vi "Teleop.vi"() -> ()   [LabVIEW 2016]
doc: "This VI is called for each TeleOp packet received from the DS where the robot is not disabled. It is often used to read from the joysticks and update I/O or to update setpoints for timed control loops. It should complete and return within 20 milliseconds or it may miss DS packets."
uses:
  <vilib>/Rock Robotics/WPI/Utilities/WPI_GetSetVariantRefNum.vi
  External/2ndContollerStatus.vi
  External/External.lvlib
panel:
  out "Angle":u16
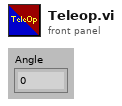
[diagram p1: front panel]
types:
  T1 = enum16{"A", "B", "X", "Y", "LB", "RB", "Back", "Start"}
  T2 = typedef "WPI_JoystickDevRef.ctl" = cluster{"Device":T3}
  T3 = typedef "WPI_JoystickDeviceEnum.ctl" = enum16{"USB 0", "USB 1", "USB 2", "USB 3", "USB 4", "USB 5"}
  T4 = typedef "WPI_RobotDriveDevRef.ctl" = cluster{"DevStatus":errorcluster, "Motors[]":T5[], "Square Inputs":bool, "Max Output":dbl}
  T5 = typedef "WPI_MotorControlDeviceRef.ctl" = cluster{"DeviceStatus":errorcluster, "Type":T6, "PWM":cluster{"PWM Channel":T7, "DeadBand":T8}, "CAN":cluster{"Device Number":u8, "SetOutput VI Ref":variant, "GetOutput VI Ref":variant, "Enable VI Ref":variant, "Disable VI Ref":variant, "Data":variant}, "Invert":bool}
  T6 = typedef "WPI_MotorControlType.ctl" = enum16{"PWM", "CAN"}
  T7 = typedef "FPGA_DIOPWMChannel.ctl" = enum8{"PWM 0", "PWM 1", "PWM 2", "PWM 3", "PWM 4", "PWM 5", "PWM 6", "PWM 7", "PWM 8", "PWM 9", "PWM MXP 0", "PWM MXP 1", "PWM MXP 2", "PWM MXP 3", "PWM MXP 4", "PWM MXP 5", "PWM MXP 6", "PWM MXP 7", "PWM MXP 8", "PWM MXP 9", "Invalid"}
  T8 = typedef "WPI_PWMDeadband.ctl" = cluster{"Name":string, "maxPositivePwm":i32, "minPositivePwm":i32, "centerPwm":i32, "maxNegativePwm":i32, "minNegativePwm":i32, "angularRange":u16}
  T9 = typedef "WPI_ServoDeviceRef.ctl" = cluster{"DeviceStatus":errorcluster, "PWM Channel":T7, "DeadBand":T8}
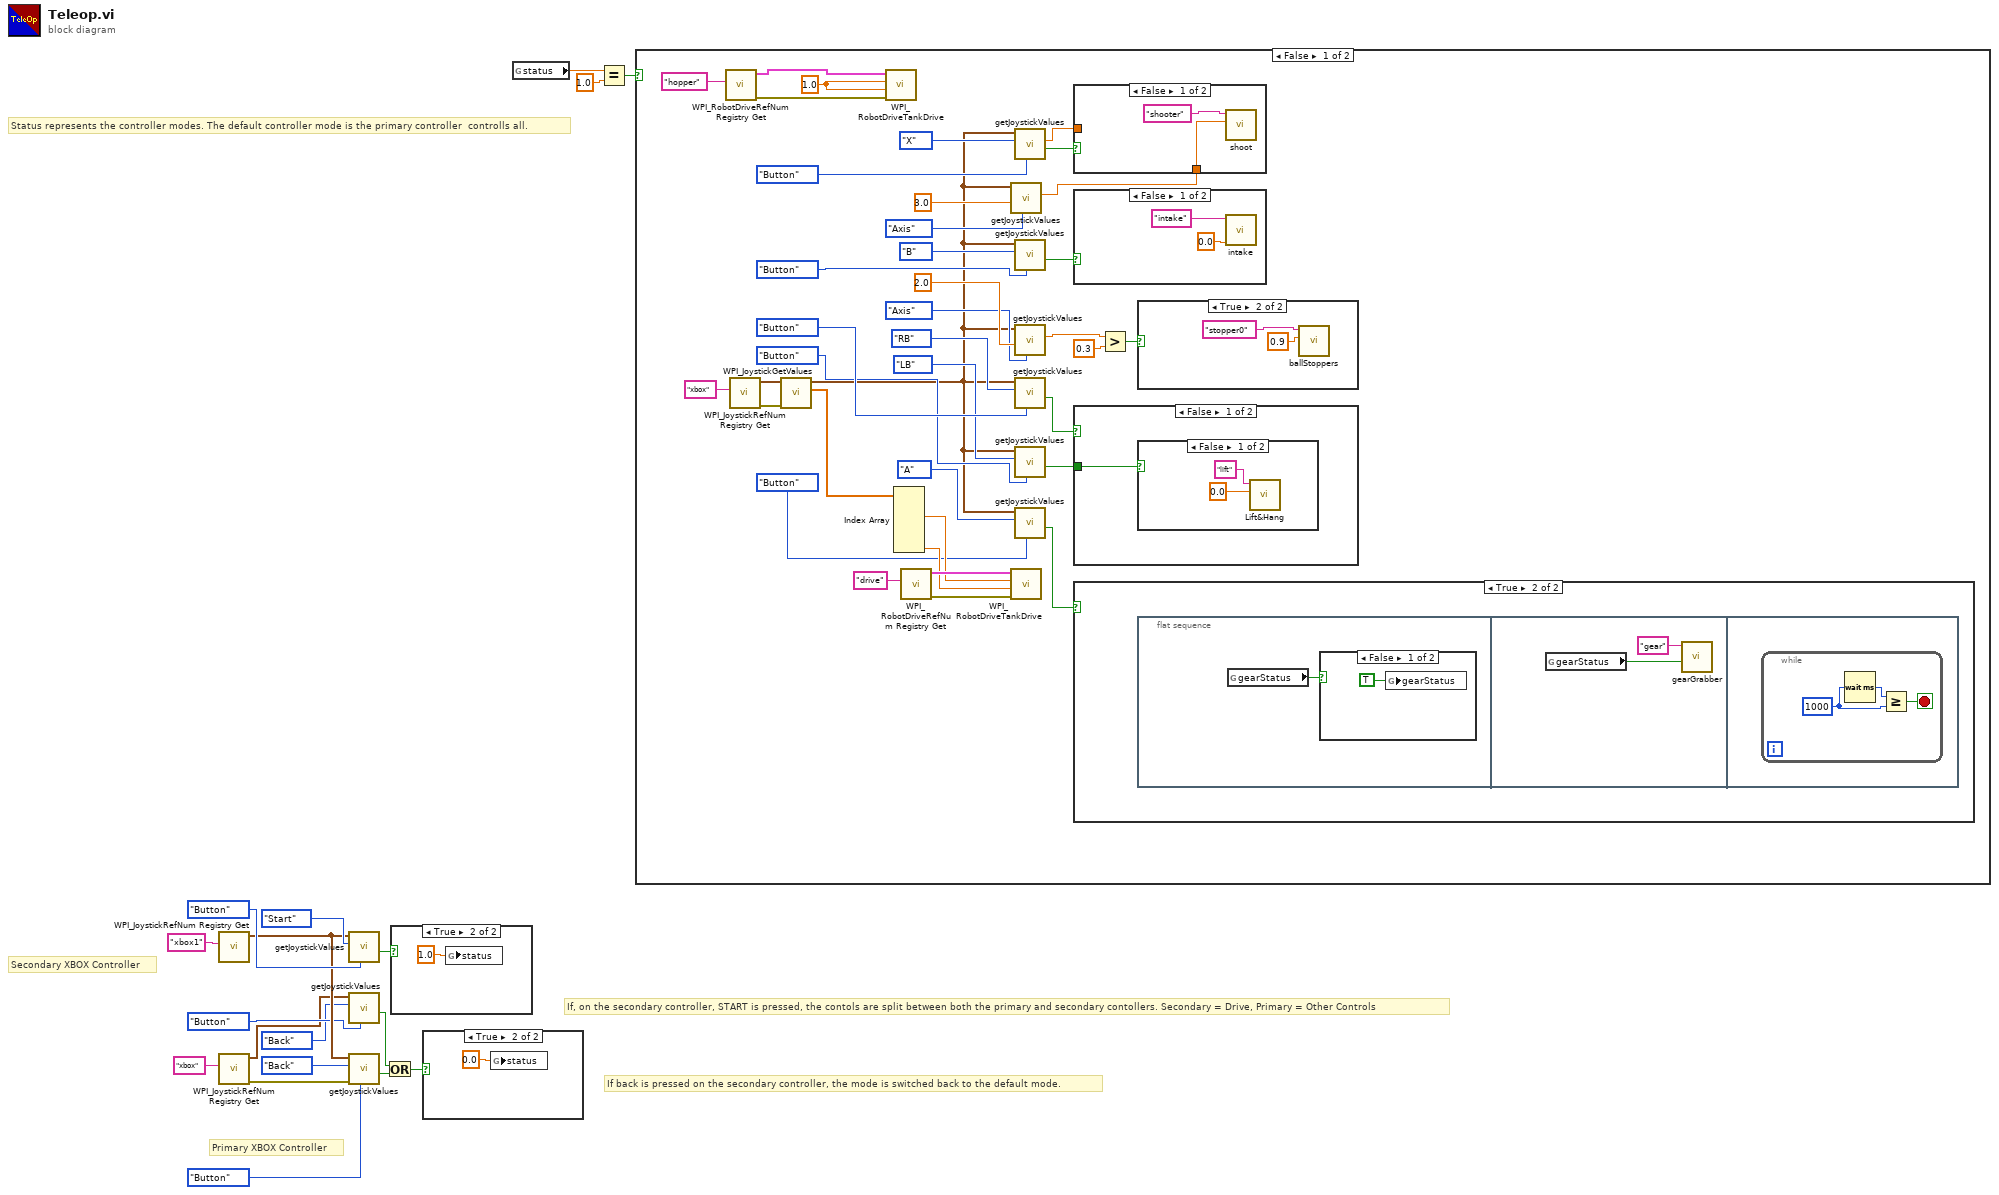
[diagram p0: block diagram]
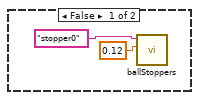
[diagram p2: hidden frame]
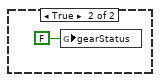
[diagram p4: hidden frame]
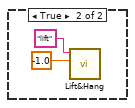
[diagram p5: hidden frame]
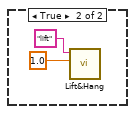
[diagram p6: hidden frame]
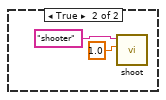
[diagram p7: hidden frame]
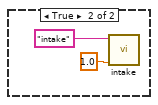
[diagram p8: hidden frame]
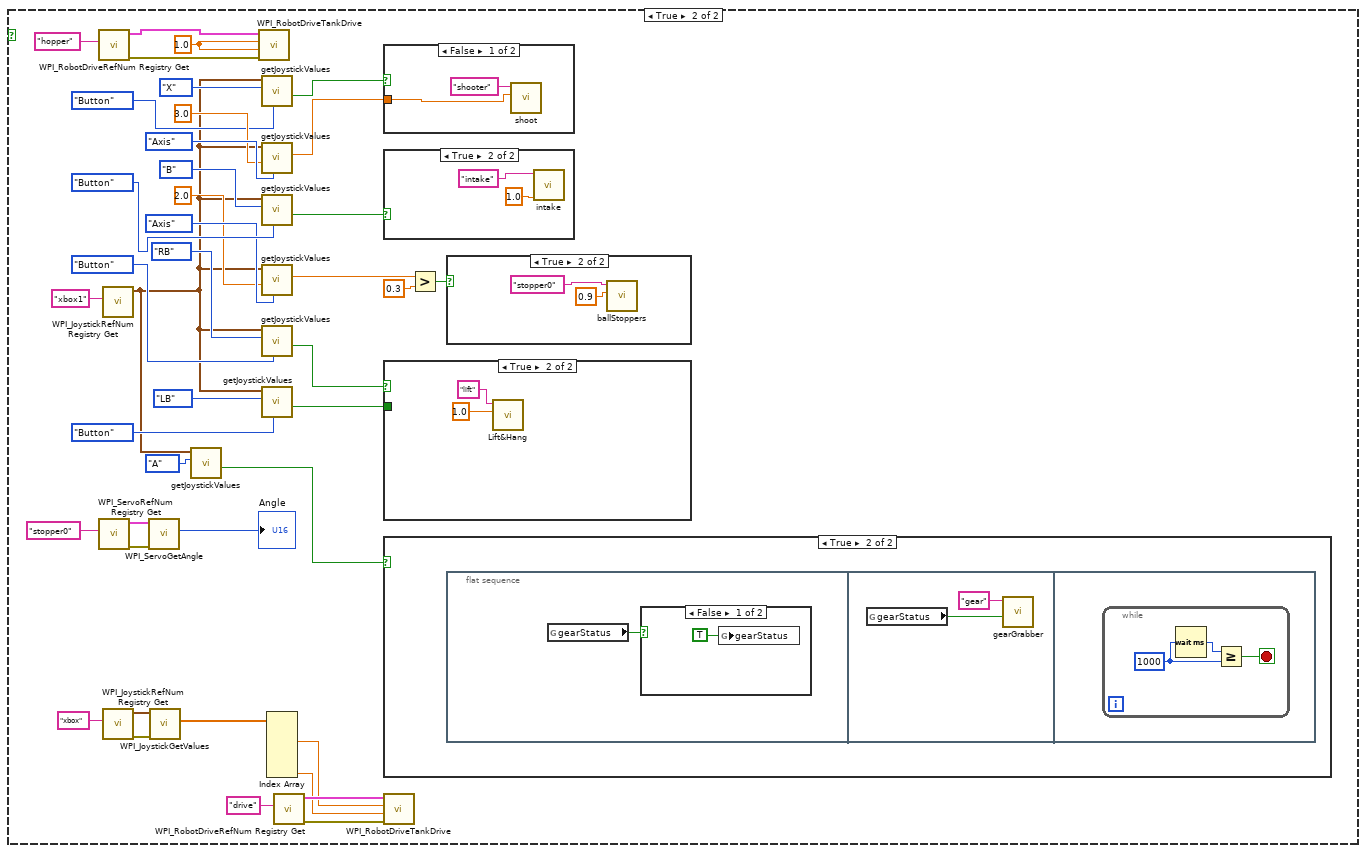
[diagram p9: hidden frame]
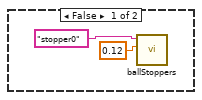
[diagram p10: hidden frame]
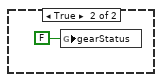
[diagram p12: hidden frame]
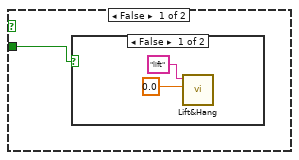
[diagram p13: hidden frame]
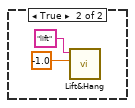
[diagram p14: hidden frame]
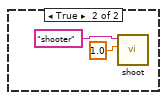
[diagram p15: hidden frame]
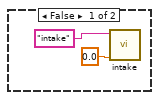
[diagram p16: hidden frame]
diagram:
  # "Secondary XBOX Controller"
  # "Primary XBOX Controller"
  # "If back is pressed on the secondary controller, the mode is switched back to the default mode."
  # "If, on the secondary controller, START is pressed, the contols are split between both the primary and secondary contollers. Secondary = Drive, Primary = Other Controls"
  # "Status represents the controller modes. The default controller mode is the primary controller  controlls all."
  n1 = call <vilib>:"WPI_JoystickRefNum Registry Get.vi"("refnum name"="xbox1" ("xbox1")) -> ("JoystickDevRef"=w13:T2)  [unwired: 9 in, 1 out]
  n2 = call <vilib>:"WPI_JoystickRefNum Registry Get.vi"("refnum name"="xbox" ("xbox")) -> ("error out"=w12:errorcluster, "JoystickDevRef"=w2:T2)  [unwired: 9 in]
  n3 = call "getJoystickValues.vi"("Mode"=enum16{"Axis", "Button"}."Button", "buttonType"=T1."Start", "JoystickDevRef"=w13) -> ("Button Pressed"=w5:bool)  [unwired: 5 in, 3 out]
  n4 = call "getJoystickValues.vi"("Mode"=enum16{"Axis", "Button"}."Button", "buttonType"=T1."Back", "JoystickDevRef"=w2) -> ("Button Pressed"=w3:bool)  [unwired: 5 in, 3 out]
  n5 = call "getJoystickValues.vi"("Mode"=enum16{"Axis", "Button"}."Button", "error in (no error)"=w12, "buttonType"=T1."Back", "JoystickDevRef"=w13) -> ("Button Pressed"=w4:bool)  [unwired: 4 in, 3 out]
  n6 = Or(x=w3, y=w4) -> (x .or. y?=w1:bool)
  n7 = case shown="True" w5 {
    frame False {
    }
    frame True {
      n8 = global write "2ndContollerStatus.vi" "status"(1.0 ("status")) -> ()
    }
  }
  n9 = case shown="True" w1 {
    frame False {
    }
    frame True {
      n10 = global write "2ndContollerStatus.vi" "status"(0.0 ("status")) -> ()
    }
  }
  n11 = global read "2ndContollerStatus.vi" "status"() -> (w11:dbl)
  n12 = Equal?(x=w11, y=1.0) -> (x = y?=w8:bool)
  n13 = case shown="False" w8 {
    frame False {
      w33 = 1.0 ("Left axis value")
      n14 = call <vilib>:"WPI_RobotDriveRefNum Registry Get.vi"("refnum name"="hopper") -> ("error out"=w35:errorcluster, "RobotDriveDevRef"=w36:T4)  [unwired: 9 in]
      n15 = call <vilib>:"WPI_JoystickRefNum Registry Get.vi"("refnum name"="xbox") -> ("error out"=w44:errorcluster, "JoystickDevRef"=w43:T2)  [unwired: 9 in]
      n16 = call <vilib>:"WPI_JoystickGetValues.vi"("error in (no error)"=w44, "JoystickDevRef"=w43) -> ("Axes"=w42:dbl[], "JoystickDevRef"=w24:T2)  [unwired: 5 in, 3 out]
      n17 = call <vilib>:"WPI_RobotDriveTankDrive.vi"("error in (no error)"=w35, "Right axis value"=w33, "Left axis value"=w33, "RobotDriveDevRef"=w36) -> ()  [unwired: 5 in, 3 out]
      n18 = Index Array(array=w42) -> (element #2=w40:dbl, element #6=w39:dbl)  [unwired: 6 in, 4 out]
      n19 = call <vilib>:"WPI_RobotDriveRefNum Registry Get.vi"("refnum name"="drive") -> ("error out"=w45:errorcluster, "RobotDriveDevRef"=w46:T4)  [unwired: 9 in]
      n20 = call "getJoystickValues.vi"("Mode"=enum16{"Axis", "Button"}."Axis", "Axis"=3.0, "JoystickDevRef"=w24) -> ("Value"=w21:dbl)  [unwired: 5 in, 3 out]
      n21 = call <vilib>:"WPI_RobotDriveTankDrive.vi"("error in (no error)"=w45, "Right axis value"=w39, "Left axis value"=w40, "RobotDriveDevRef"=w46) -> ()  [unwired: 5 in, 3 out]
      n22 = call "getJoystickValues.vi"("Mode"=enum16{"Axis", "Button"}."Button", "buttonType"=T1."X", "JoystickDevRef"=w24) -> ("Button Pressed"=w30:bool, "Value"=w22:dbl)  [unwired: 5 in, 2 out]
      n23 = call "getJoystickValues.vi"("Mode"=enum16{"Axis", "Button"}."Button", "buttonType"=T1."B", "JoystickDevRef"=w24) -> ("Button Pressed"=w58:bool)  [unwired: 5 in, 3 out]
      n24 = call "getJoystickValues.vi"("Mode"=enum16{"Axis", "Button"}."Axis", "Axis"=2.0, "JoystickDevRef"=w24) -> ("Value"=w23:dbl)  [unwired: 5 in, 3 out]
      n25 = call "getJoystickValues.vi"("Mode"=enum16{"Axis", "Button"}."Button", "buttonType"=T1."RB", "JoystickDevRef"=w24) -> ("Button Pressed"=w53:bool)  [unwired: 5 in, 3 out]
      n26 = call "getJoystickValues.vi"("Mode"=enum16{"Axis", "Button"}."Button", "buttonType"=T1."LB", "JoystickDevRef"=w24) -> ("Button Pressed"=w48:bool)  [unwired: 5 in, 3 out]
      n27 = call "getJoystickValues.vi"("Mode"=enum16{"Axis", "Button"}."Button", "buttonType"=T1."A", "JoystickDevRef"=w24) -> ("Button Pressed"=w38:bool)  [unwired: 5 in, 3 out]
      n28 = case shown="False" w30 {
        tunnel: w22 -> [_ _]
        tunnel: w21 -> [w78 _]
        frame False {
          n29 = call "shoot.vi"("Motor Power"=w78, "refnum name"="shooter") -> ()  [unwired: 9 in, 1 out]
        }
        frame True {
          n30 = call "shoot.vi"("Motor Power"=1.0, "refnum name"="shooter") -> ()  [unwired: 9 in, 1 out]
        }
      }
      n31 = case shown="False" w58 {
        frame False {
          n32 = call "intake.vi"("intakeSpeed"=0.0, "intake"="intake") -> ()  [unwired: 9 in, 1 out]
        }
        frame True {
          n33 = call "intake.vi"("intakeSpeed"=1.0, "intake"="intake") -> ()  [unwired: 9 in, 1 out]
        }
      }
      n34 = case shown="False" w53 {
        tunnel: w48 -> [w71 _]
        frame False {
          n35 = case shown="False" w71 {
            frame False {
              n36 = call "Lift&Hang.vi"("status"=0.0, "refnum name"="lift" ("lift")) -> ()  [unwired: 9 in, 1 out]
            }
            frame True {
              n37 = call "Lift&Hang.vi"("status"=-1.0, "refnum name"="lift" ("lift")) -> ()  [unwired: 9 in, 1 out]
            }
          }
        }
        frame True {
          n38 = call "Lift&Hang.vi"("status"=1.0, "refnum name"="lift" ("lift")) -> ()  [unwired: 9 in, 1 out]
        }
      }
      n39 = case shown="True" w38 {
        frame False {
        }
        frame True {
          n40 = flat-sequence {
            frame #0 {
              n41 = global read "2ndContollerStatus.vi" "gearStatus"() -> (w63:bool)
              n42 = case shown="False" w63 {
                frame False {
                  n43 = global write "2ndContollerStatus.vi" "gearStatus"(TRUE ("gearStatus")) -> ()
                }
                frame True {
                  n44 = global write "2ndContollerStatus.vi" "gearStatus"(FALSE ("gearStatus")) -> ()
                }
              }
            }
            frame #1 {
              n45 = global read "2ndContollerStatus.vi" "gearStatus"() -> (w66:bool)
              n46 = call "gearGrabber.vi"("gearStatus"=w66, "gear"="gear") -> ()  [unwired: 9 in, 1 out]
            }
            frame #2 {
              n47 = while {
                stop <- w70 stop-if-true
                w68 = u32 1000 ("milliseconds to wait")
                n48 = Wait (ms)(milliseconds to wait=w68) -> (millisecond timer value=w69:u32)
                n49 = Greater Or Equal?(x=w69, y=w68) -> (x >= y?=w70:bool)
              }
            }
          }
        }
      }
      n50 = Greater?(x=w23, y=0.3) -> (0:w27:bool)
      n51 = case shown="True" w27 {
        frame False {
          n52 = call "ballStoppers.vi"("stopperValue"=0.12, "stopper1 or stopper0"="stopper0") -> ()  [unwired: 9 in, 1 out]
        }
        frame True {
          n53 = call "ballStoppers.vi"("stopperValue"=0.9, "stopper1 or stopper0"="stopper0") -> ()  [unwired: 9 in, 1 out]
        }
      }
    }
    frame True {
      w100 = 1.0 ("Left axis value")
      n54 = call <vilib>:"WPI_RobotDriveRefNum Registry Get.vi"("refnum name"="hopper") -> ("error out"=w102:errorcluster, "RobotDriveDevRef"=w103:T4)  [unwired: 9 in]
      n55 = call <vilib>:"WPI_ServoRefNum Registry Get.vi"("refnum name"="stopper0") -> ("error out"=w88:errorcluster, "ServoDeviceRef"=w89:T9)  [unwired: 9 in]
      n56 = call <vilib>:"WPI_JoystickRefNum Registry Get.vi"("refnum name"="xbox1") -> ("JoystickDevRef"=w90:T2)  [unwired: 9 in, 1 out]
      n57 = call <vilib>:"WPI_JoystickRefNum Registry Get.vi"("refnum name"="xbox") -> ("error out"=w111:errorcluster, "JoystickDevRef"=w110:T2)  [unwired: 9 in]
      n58 = call <vilib>:"WPI_ServoGetAngle.vi"("ServoDeviceRef"=w89, "error in (no error)"=w88) -> ("Angle"=→"Angle":u16)  [unwired: 6 in, 2 out]
      n59 = call <vilib>:"WPI_JoystickGetValues.vi"("error in (no error)"=w111, "JoystickDevRef"=w110) -> ("Axes"=w109:dbl[])  [unwired: 5 in, 4 out]
      n60 = call "getJoystickValues.vi"("buttonType"=T1."A", "JoystickDevRef"=w90) -> ("Button Pressed"=w105:bool)  [unwired: 6 in, 3 out]
      n61 = call <vilib>:"WPI_RobotDriveTankDrive.vi"("error in (no error)"=w102, "Right axis value"=w100, "Left axis value"=w100, "RobotDriveDevRef"=w103) -> ()  [unwired: 5 in, 3 out]
      n62 = call "getJoystickValues.vi"("Mode"=enum16{"Axis", "Button"}."Button", "buttonType"=T1."X", "JoystickDevRef"=w90) -> ("Button Pressed"=w96:bool)  [unwired: 5 in, 3 out]
      n63 = call "getJoystickValues.vi"("Mode"=enum16{"Axis", "Button"}."Axis", "Axis"=3.0, "JoystickDevRef"=w90) -> ("Value"=w99:dbl)  [unwired: 5 in, 3 out]
      n64 = call "getJoystickValues.vi"("Mode"=enum16{"Axis", "Button"}."Button", "buttonType"=T1."B", "JoystickDevRef"=w90) -> ("Button Pressed"=w126:bool)  [unwired: 5 in, 3 out]
      n65 = call "getJoystickValues.vi"("Mode"=enum16{"Axis", "Button"}."Axis", "Axis"=2.0, "JoystickDevRef"=w90) -> ("Value"=w91:dbl)  [unwired: 5 in, 3 out]
      n66 = call "getJoystickValues.vi"("Mode"=enum16{"Axis", "Button"}."Button", "buttonType"=T1."RB", "JoystickDevRef"=w90) -> ("Button Pressed"=w120:bool)  [unwired: 5 in, 3 out]
      n67 = call "getJoystickValues.vi"("Mode"=enum16{"Axis", "Button"}."Button", "buttonType"=T1."LB", "JoystickDevRef"=w90) -> ("Button Pressed"=w115:bool)  [unwired: 5 in, 3 out]
      n68 = Index Array(array=w109) -> (element #2=w107:dbl, element #6=w106:dbl)  [unwired: 6 in, 4 out]
      n69 = call <vilib>:"WPI_RobotDriveRefNum Registry Get.vi"("refnum name"="drive") -> ("error out"=w112:errorcluster, "RobotDriveDevRef"=w113:T4)  [unwired: 9 in]
      n70 = case shown="False" w96 {
        tunnel: w99 -> [w146 _]
        frame False {
          n71 = call "shoot.vi"("Motor Power"=w146, "refnum name"="shooter") -> ()  [unwired: 9 in, 1 out]
        }
        frame True {
          n72 = call "shoot.vi"("Motor Power"=1.0, "refnum name"="shooter") -> ()  [unwired: 9 in, 1 out]
        }
      }
      n73 = case shown="True" w126 {
        frame False {
          n74 = call "intake.vi"("intakeSpeed"=0.0, "intake"="intake") -> ()  [unwired: 9 in, 1 out]
        }
        frame True {
          n75 = call "intake.vi"("intakeSpeed"=1.0, "intake"="intake") -> ()  [unwired: 9 in, 1 out]
        }
      }
      n76 = case shown="True" w120 {
        tunnel: w115 -> [w139 _]
        frame False {
          n77 = case shown="False" w139 {
            frame False {
              n78 = call "Lift&Hang.vi"("status"=0.0, "refnum name"="lift" ("lift")) -> ()  [unwired: 9 in, 1 out]
            }
            frame True {
              n79 = call "Lift&Hang.vi"("status"=-1.0, "refnum name"="lift" ("lift")) -> ()  [unwired: 9 in, 1 out]
            }
          }
        }
        frame True {
          n80 = call "Lift&Hang.vi"("status"=1.0, "refnum name"="lift" ("lift")) -> ()  [unwired: 9 in, 1 out]
        }
      }
      n81 = case shown="True" w105 {
        frame False {
        }
        frame True {
          n82 = flat-sequence {
            frame #0 {
              n83 = global read "2ndContollerStatus.vi" "gearStatus"() -> (w131:bool)
              n84 = case shown="False" w131 {
                frame False {
                  n85 = global write "2ndContollerStatus.vi" "gearStatus"(TRUE ("gearStatus")) -> ()
                }
                frame True {
                  n86 = global write "2ndContollerStatus.vi" "gearStatus"(FALSE ("gearStatus")) -> ()
                }
              }
            }
            frame #1 {
              n87 = global read "2ndContollerStatus.vi" "gearStatus"() -> (w134:bool)
              n88 = call "gearGrabber.vi"("gearStatus"=w134, "gear"="gear") -> ()  [unwired: 9 in, 1 out]
            }
            frame #2 {
              n89 = while {
                stop <- w138 stop-if-true
                w136 = u32 1000 ("milliseconds to wait")
                n90 = Wait (ms)(milliseconds to wait=w136) -> (millisecond timer value=w137:u32)
                n91 = Greater Or Equal?(x=w137, y=w136) -> (x >= y?=w138:bool)
              }
            }
          }
        }
      }
      n92 = call <vilib>:"WPI_RobotDriveTankDrive.vi"("error in (no error)"=w112, "Right axis value"=w106, "Left axis value"=w107, "RobotDriveDevRef"=w113) -> ()  [unwired: 5 in, 3 out]
      n93 = Greater?(x=w91, y=0.3) -> (0:w94:bool)
      n94 = case shown="True" w94 {
        frame False {
          n95 = call "ballStoppers.vi"("stopperValue"=0.12, "stopper1 or stopper0"="stopper0") -> ()  [unwired: 9 in, 1 out]
        }
        frame True {
          n96 = call "ballStoppers.vi"("stopperValue"=0.9, "stopper1 or stopper0"="stopper0") -> ()  [unwired: 9 in, 1 out]
        }
      }
    }
  }
